vi "Format Channel Names - Crosstalk.vi"(10 "names in":string[](array[string])) -> (2 "names out":string[](array[string]))   [LabVIEW 2023]
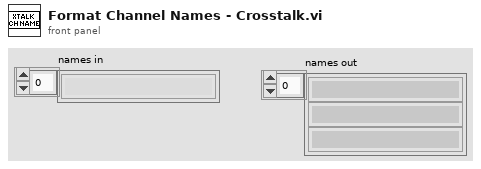
[diagram p1: front panel]
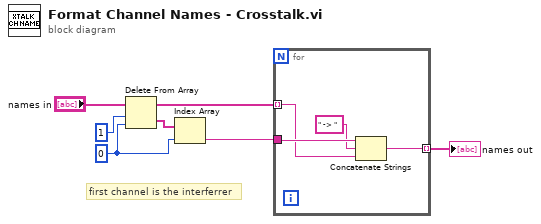
[diagram p0: block diagram]
diagram:
  w4 = 0 ("index")
  # "first channel is the interferrer"
  n1 = Delete From Array(array="names in", length=1, index=w4) -> (deleted portion=w5:string[], array with subset deleted=w3:string[])
  n2 = Index Array(array=w5, index=w4) -> (element=w2:string)
  n3 = for {
    tunnel: w3 -> [w9] mode=indexing
    tunnel: w2 -> [w11]
    tunnel: [w8] -> w1 mode=indexing
    n4 = Concatenate Strings(w11, " -> " ("string"), w9) -> (w8:string)
  }
  "names out" <- w1
